vi "Lab2-InstructorHint-Calc-DisplayOnly.vi"() -> ()   [LabVIEW 2018]
panel:
  out "DegFlag":bool
  in  "Tab Control":enum32{"Calculator", "Settings", "Debug"}(tab)
  in  "Calc Pad Cluster":T1
  out "Calc Display":string
  out "Mode":string
  in  "ButtonPropertiesArray":T2(array[cluster])=[{"On/off"=FALSE, "Character"="C", "Op?"=FALSE}, {"On/off"=FALSE, "Character"="sin", "Op?"=FALSE}, {"On/off"=FALSE, "Character"="cos", "Op?"=FALSE}, {"On/off"=FALSE, "Character"="Del", "Op?"=FALSE}, {"On/off"=FALSE, "Character"="+", "Op?"=FALSE}, {"On/off"=FALSE, "Character"="7", "Op?"=FALSE}, {"On/off"=FALSE, "Character"="8", "Op?"=FALSE}, {"On/off"=FALSE, "Character"="9", "Op?"=FALSE}, {"On/off"=FALSE, "Character"="-", "Op?"=FALSE}, {"On/off"=FALSE, "Character"="4", "Op?"=FALSE}, {"On/off"=FALSE, "Character"="5", "Op?"=FALSE}, {"On/off"=FALSE, "Character"="6", "Op?"=FALSE}, {"On/off"=FALSE, "Character"="*", "Op?"=FALSE}, {"On/off"=FALSE, "Character"="1", "Op?"=FALSE}, {"On/off"=FALSE, "Character"="2", "Op?"=FALSE}, {"On/off"=FALSE, "Character"="3", "Op?"=FALSE}, {"On/off"=FALSE, "Character"="/", "Op?"=FALSE}, {"On/off"=FALSE, "Character"="(", "Op?"=FALSE}, {"On/off"=FALSE, "Character"=")", "Op?"=FALSE}, {"On/off"=FALSE, "Character"="=", "Op?"=FALSE}, {"On/off"=FALSE, "Character"=".", "Op?"=FALSE}, {"On/off"=FALSE, "Character"="Equation", "Op?"=FALSE}, {"On/off"=FALSE, "Character"="^", "Op?"=FALSE}, {"On/off"=FALSE, "Character"="0", "Op?"=FALSE}, {"On/off"=FALSE, "Character"="tan", "Op?"=FALSE}, {"On/off"=FALSE, "Character"="exit", "Op?"=FALSE}, {"On/off"=FALSE, "Character"="Rad", "Op?"=FALSE}]
  out "ButtonIndex":i32[](array[numeric])
  out "ButtonChars":string[](array[string])
  out "KeyPressedStatus":bool[](array[boolean])
  out "c":dbl
  out "b":dbl
  out "a":dbl
  out "EqState":dbl
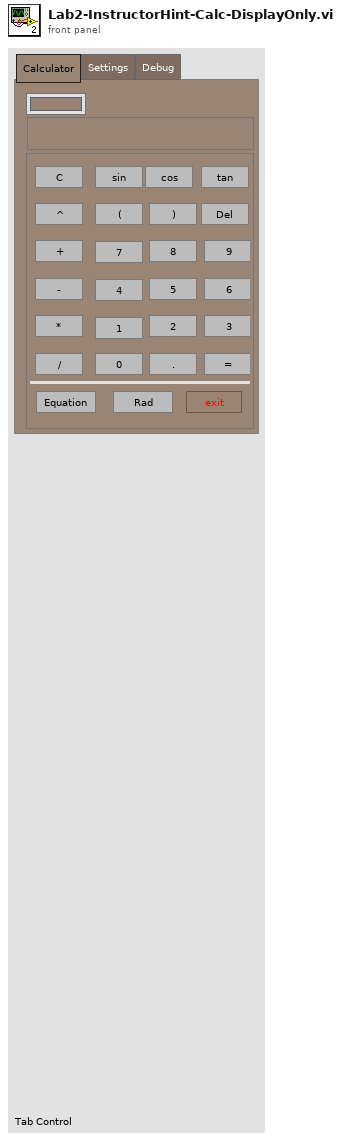
[diagram p1: front panel]
types:
  T1 = cluster{"B 0":bool, "B 1":bool, "B 2":bool, "B 3":bool, "B 4":bool, "B 5":bool, "B 6":bool, "B 7":bool, "B 8":bool, "B 9":bool, "B 10":bool, "B 11":bool, "B 12":bool, "B 13":bool, "B 14":bool, "B 15":bool, "B 16":bool, "B 17":bool, "B 18":bool, "B 19":bool, "B 20":bool, "B 21":bool, "B 22":bool, "B 23":bool, "B 24":bool, "Exit":bool, "B 25":bool}
  T2 = cluster{"On/off":bool, "Character":string, "Op?":bool}[]
  T3 = cluster{"On/off":bool, "Character":string, "Op?":bool}
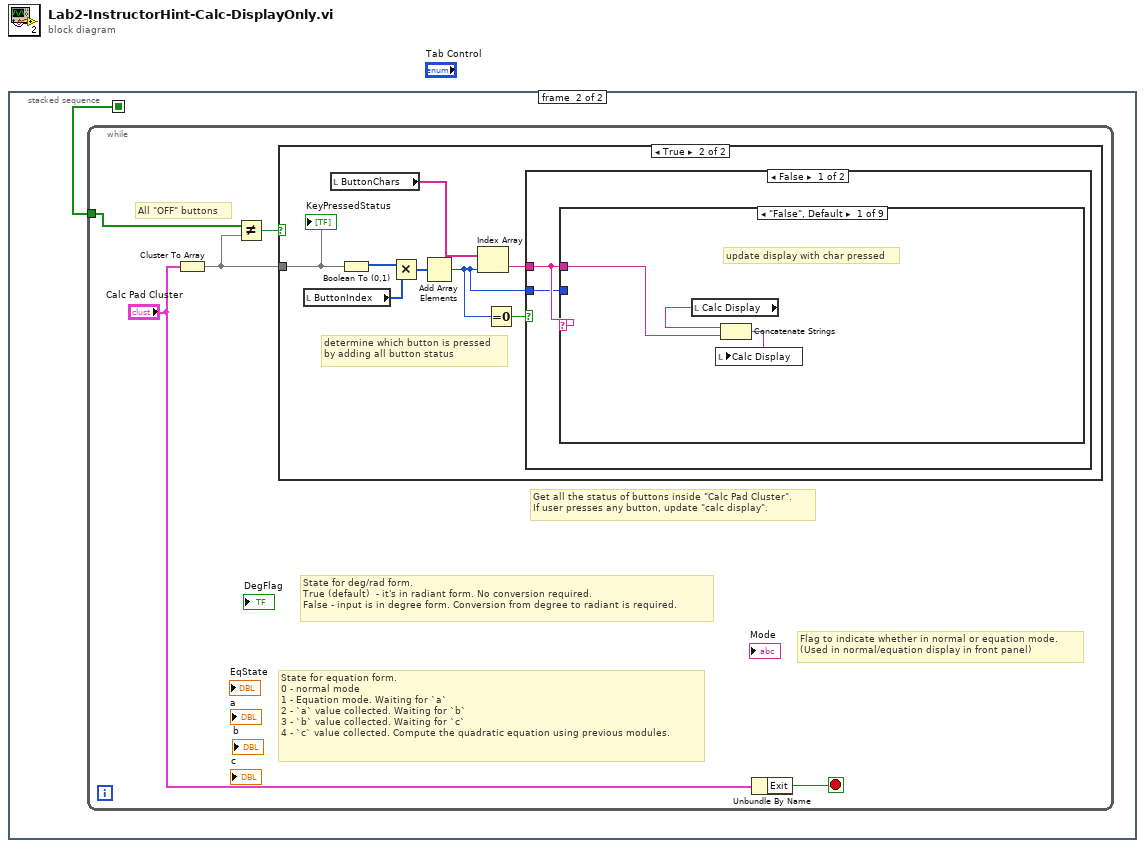
[diagram p0: block diagram]
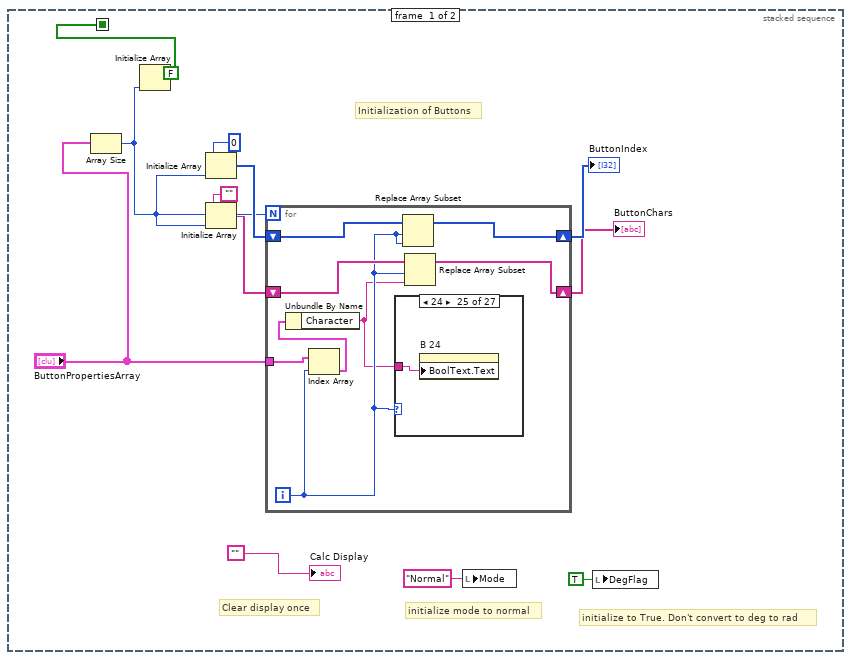
[diagram p2: hidden frame]
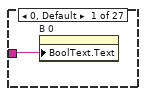
[diagram p3: hidden frame]
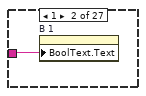
[diagram p4: hidden frame]
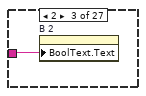
[diagram p5: hidden frame]
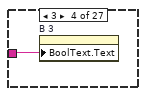
[diagram p6: hidden frame]
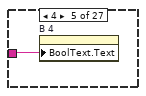
[diagram p7: hidden frame]
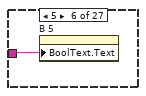
[diagram p8: hidden frame]
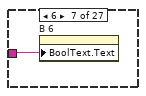
[diagram p9: hidden frame]
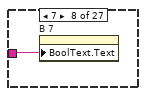
[diagram p10: hidden frame]
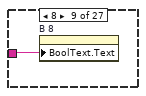
[diagram p11: hidden frame]
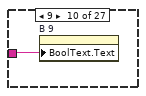
[diagram p12: hidden frame]
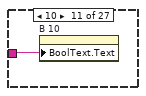
[diagram p13: hidden frame]
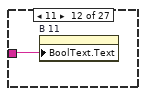
[diagram p14: hidden frame]
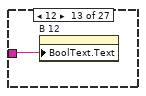
[diagram p15: hidden frame]
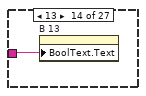
[diagram p16: hidden frame]
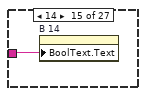
[diagram p17: hidden frame]
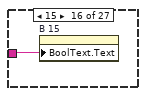
[diagram p18: hidden frame]
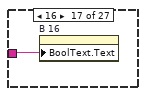
[diagram p19: hidden frame]
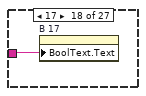
[diagram p20: hidden frame]
diagram:
  n1 = stacked-sequence {
    seq-local: [w12 _] -> [_ w49]
    frame #0 {
      # "initialize to True. Don't convert to deg to rad"
      # "initialize mode to normal"
      # "Clear display once"
      # "Initialization of Buttons"
      n2 = Array Size(array="ButtonPropertiesArray") -> (size(s)=w6:i32)
      n3 = Initialize Array(FALSE, w6) -> (w12:bool[])
      n4 = Initialize Array(0, w6) -> (w9:i32[])
      n5 = Initialize Array("", w6) -> (w5:string[])
      n6 = for {
        N: w6 -> [_]
        tunnel: "ButtonPropertiesArray" -> [w17]
        shift-right: [w20] -> w8
        shift-left: w9 -> [w21]
        shift-right: [w16] -> w4
        shift-left: w5 -> [w19]
        i -> [w15]
        n7 = Index Array(array=w17, index=w15) -> (element=w18:T3)
        n8 = Unbundle By Name(w18) -> ("Character"=w14:string)
        n9 = case shown="24" w15 {
          tunnel: w14 -> [w22 w23 w24 w25 w26 w27 w28 w29 w30 w31 w32 w33 w34 w35 w36 w37 w38 w39 w40 w41 w42 w43 w44 w45 w46 w47 w48]
          frame 0, Default {
            n10 = property on="B 0" class="Bool"("BoolText.Text"=w22) -> ()  [unwired: 2 in, 2 out]
          }
          frame 1 {
            n11 = property on="B 1" class="Bool"("BoolText.Text"=w23) -> ()  [unwired: 2 in, 2 out]
          }
          frame 2 {
            n12 = property on="B 2" class="Bool"("BoolText.Text"=w24) -> ()  [unwired: 2 in, 2 out]
          }
          frame 3 {
            n13 = property on="B 3" class="Bool"("BoolText.Text"=w25) -> ()  [unwired: 2 in, 2 out]
          }
          frame 4 {
            n14 = property on="B 4" class="Bool"("BoolText.Text"=w26) -> ()  [unwired: 2 in, 2 out]
          }
          frame 5 {
            n15 = property on="B 5" class="Bool"("BoolText.Text"=w27) -> ()  [unwired: 2 in, 2 out]
          }
          frame 6 {
            n16 = property on="B 6" class="Bool"("BoolText.Text"=w28) -> ()  [unwired: 2 in, 2 out]
          }
          frame 7 {
            n17 = property on="B 7" class="Bool"("BoolText.Text"=w29) -> ()  [unwired: 2 in, 2 out]
          }
          frame 8 {
            n18 = property on="B 8" class="Bool"("BoolText.Text"=w30) -> ()  [unwired: 2 in, 2 out]
          }
          frame 9 {
            n19 = property on="B 9" class="Bool"("BoolText.Text"=w31) -> ()  [unwired: 2 in, 2 out]
          }
          frame 10 {
            n20 = property on="B 10" class="Bool"("BoolText.Text"=w32) -> ()  [unwired: 2 in, 2 out]
          }
          frame 11 {
            n21 = property on="B 11" class="Bool"("BoolText.Text"=w33) -> ()  [unwired: 2 in, 2 out]
          }
          frame 12 {
            n22 = property on="B 12" class="Bool"("BoolText.Text"=w34) -> ()  [unwired: 2 in, 2 out]
          }
          frame 13 {
            n23 = property on="B 13" class="Bool"("BoolText.Text"=w35) -> ()  [unwired: 2 in, 2 out]
          }
          frame 14 {
            n24 = property on="B 14" class="Bool"("BoolText.Text"=w36) -> ()  [unwired: 2 in, 2 out]
          }
          frame 15 {
            n25 = property on="B 15" class="Bool"("BoolText.Text"=w37) -> ()  [unwired: 2 in, 2 out]
          }
          frame 16 {
            n26 = property on="B 16" class="Bool"("BoolText.Text"=w38) -> ()  [unwired: 2 in, 2 out]
          }
          frame 17 {
            n27 = property on="B 17" class="Bool"("BoolText.Text"=w39) -> ()  [unwired: 2 in, 2 out]
          }
          frame 18 {
            n28 = property on="B 18" class="Bool"("BoolText.Text"=w40) -> ()  [unwired: 2 in, 2 out]
          }
          frame 19 {
            n29 = property on="B 19" class="Bool"("BoolText.Text"=w41) -> ()  [unwired: 2 in, 2 out]
          }
          frame 20 {
            n30 = property on="B 20" class="Bool"("BoolText.Text"=w42) -> ()  [unwired: 2 in, 2 out]
          }
          frame 21 {
            n31 = property on="B 21" class="Bool"("BoolText.Text"=w43) -> ()  [unwired: 2 in, 2 out]
          }
          frame 22 {
            n32 = property on="B 22" class="Bool"("BoolText.Text"=w44) -> ()  [unwired: 2 in, 2 out]
          }
          frame 23 {
            n33 = property on="B 23" class="Bool"("BoolText.Text"=w45) -> ()  [unwired: 2 in, 2 out]
          }
          frame 24 {
            n34 = property on="B 24" class="Bool"("BoolText.Text"=w46) -> ()  [unwired: 2 in, 2 out]
          }
          frame 25 {
            n35 = property on="Exit" class="Bool"("BoolText.Text"=w47) -> ()  [unwired: 2 in, 2 out]
          }
          frame 26 {
            n36 = property on="B 25" class="Bool"("BoolText.Text"=w48) -> ()  [unwired: 2 in, 2 out]
          }
        }
        n37 = Replace Array Subset(array=w21, new element=w15, index=w15) -> (w20:i32[])
        n38 = Replace Array Subset(array=w19, new element=w14, index=w15) -> (w16:string[])
      }
      "ButtonIndex" <- w8
      "ButtonChars" <- w4
      n39 = local write "Mode"("Normal" ("Mode")) -> ()
      n40 = local write "DegFlag"(TRUE ("DegFlag")) -> ()
      "Calc Display" <- ""
    }
    frame #1 {
      n41 = while {
        tunnel: w49 -> [w52]
        stop <- w50 stop-if-true
        # "Flag to indicate whether in normal or equation mode.\n(Used in normal/equation display in front panel)"
        # "State for deg/rad form.\nTrue (default)  - it's in radiant form. No conversion required.\nFalse - input is in degree form. Conversion from degree to radiant is required."
        # "State for equation form. \n0 - normal mode\n1 - Equation mode. Waiting for `a`\n2 - `a` value collected. Waiting for `b`\n3 - `b` value collected. Waiting for `c`\n4 - `c` value collected. Compute the quadratic equation using previous modules."
        # "Get all the status of buttons inside \"Calc Pad Cluster\".\nIf user presses any button, update \"calc display\"."
        # "All \"OFF\" buttons"
        n42 = Cluster To Array(cluster="Calc Pad Cluster") -> (array=w53:bool[])
        n43 = Not Equal?(x=w52, y=w53) -> (x != y?=w54:bool)
        n44 = case shown="True" w54 {
          tunnel: w53 -> [_ w57]
          frame False {
            # "no button is pressed"
          }
          frame True {
            # "determine which button is pressed\nby adding all button status"
            n45 = local read "ButtonIndex"() -> (w61:i32[])
            n46 = local read "ButtonChars"() -> (w59:string[])
            n47 = Boolean To (0,1)(Boolean=w57) -> (0, 1=w62:i16[])
            n48 = Multiply(x=w62, y=w61) -> (x*y=w60:i32[])
            n49 = Add Array Elements(numeric array=w60) -> (sum=w55:i32)
            n50 = Index Array(array=w59, index=w55) -> (element=w58:string)
            n51 = Equal To 0?(x=w55) -> (x = 0?=w56:bool)
            n52 = case shown="False" w56 {
              tunnel: w58 -> [w64 _]
              tunnel: w55 -> [w63 _]
              frame False {
                n53 = case shown="\"False\", Default" w64 {
                  tunnel: w64 -> [w66 _ _ w101 w104 w108 _ _ _]
                  tunnel: w63 -> [_ _ _ _ _ _ _ w116 w122]
                  frame "False", Default {
                    # "update display with char pressed"
                    n54 = local read "Calc Display"() -> (w67:string)
                    n55 = Concatenate Strings(w67, w66) -> (w65:string)
                    n56 = local write "Calc Display"(w65) -> ()
                  }
                  frame "=" {
                    n57 = local read "EqState"() -> (w68:dbl)
                    n58 = case shown="3" w68 {
                      frame 0, Default {
                        # "DegFlag is used to indicate whether \ncurrent string is in degree or radiant\nform"
                        n59 = local read "DegFlag"() -> (w70:bool)
                        n60 = local read "Calc Display"() -> (w71:string)
                        n61 = call "CalculateInputString_v2.vi"("Rad"=w70, "InputString"=w71) -> ("result"=w69:dbl)
                        n62 = Number To Fractional String(number=w69) -> (F-format string=w72:string)  [unwired: 3 in]
                        n63 = local write "Calc Display"(w72) -> ()
                      }
                      frame 1 {
                        n64 = flat-sequence {
                          frame #0 {
                            n65 = local read "Calc Display"() -> (w75:string)
                            n66 = Fract/Exp String To Number(string=w75) -> (number=w74:dbl)  [unwired: 3 in, 1 out]
                            n67 = local write "a"(w74) -> ()
                            n68 = local write "EqState"(2.0 ("EqFlag")) -> ()
                          }
                          frame #1 {
                            n69 = local write "Calc Display"("" ("Calc Display")) -> ()
                          }
                        }
                      }
                      frame 2 {
                        n70 = flat-sequence {
                          frame #0 {
                            n71 = local read "Calc Display"() -> (w79:string)
                            n72 = Fract/Exp String To Number(string=w79) -> (number=w78:dbl)  [unwired: 3 in, 1 out]
                            n73 = local write "b"(w78) -> ()
                            n74 = local write "EqState"(3.0 ("EqFlag")) -> ()
                          }
                          frame #1 {
                            n75 = local write "Calc Display"("" ("Calc Display")) -> ()
                          }
                        }
                      }
                      frame 3 {
                        # "change mode back\nto normal"
                        n76 = local write "Mode"("normal" ("Mode")) -> ()
                        n77 = local read "Calc Display"() -> (w94:string)
                        n78 = Fract/Exp String To Number(string=w94) -> (number=w93:dbl)  [unwired: 3 in, 1 out]
                        n79 = local write "c"(w93) -> ()
                        n80 = local read "c"() -> (w84:dbl)
                        n81 = local read "b"() -> (w85:dbl)
                        n82 = local read "a"() -> (w86:dbl)
                        n83 = local write "EqState"(0.0 ("EqFlag")) -> ()
                        n84 = call "quadratic_eq_solve.vi"("C"=w84, "B"=w85, "A"=w86) -> ("x2"=w82:dbl, "x1"=w83:dbl)
                        n85 = Number To Fractional String(number=w83) -> (F-format string=w90:string)  [unwired: 3 in]
                        n86 = Number To Fractional String(number=w82) -> (F-format string=w89:string)  [unwired: 3 in]
                        n87 = Concatenate Strings("x1=" ("string"), w90, "x2=" ("string"), w89) -> (w87:string)
                        n88 = local write "Calc Display"(w87) -> ()
                      }
                    }
                  }
                  frame "Del" {
                    n89 = local read "Calc Display"() -> (w98:string)
                    n90 = String Length(string=w98) -> (length=w97:i32)
                    n91 = Decrement(x=w97) -> (x-1=w96:i32)
                    n92 = Replace Substring(2:w96, 5:w98) -> (0:w95:string)  [unwired: 2 in, 1 out]
                    n93 = local write "Calc Display"(w95) -> ()
                  }
                  frame "sin" {
                    n94 = local read "Calc Display"() -> (w102:string)
                    n95 = Concatenate Strings(w102, w101, "(" ("string")) -> (w99:string)
                    n96 = local write "Calc Display"(w99) -> ()
                  }
                  frame "cos" {
                    n97 = local read "Calc Display"() -> (w105:string)
                    n98 = Concatenate Strings(w105, w104, "(" ("string")) -> (w103:string)
                    n99 = local write "Calc Display"(w103) -> ()
                  }
                  frame "tan" {
                    n100 = local read "Calc Display"() -> (w109:string)
                    n101 = Concatenate Strings(w109, w108, "(" ("string")) -> (w107:string)
                    n102 = local write "Calc Display"(w107) -> ()
                  }
                  frame "Equation" {
                    n103 = local write "Calc Display"("" ("Calc Display")) -> ()
                    n104 = local write "EqState"(1.0 ("EqFlag")) -> ()
                    n105 = local write "Mode"("Equation" ("Mode")) -> ()
                  }
                  frame "Rad" {
                    w115 = "Deg" ("Boolean Text.Text")
                    # "Rad button is clicked. Change to Deg"
                    n106 = local write "DegFlag"(FALSE ("DegFlag")) -> ()
                    n107 = property on="B 25" class="Bool"("BoolText.Text"=w115) -> ()  [unwired: 2 in, 2 out]
                    n108 = local read "ButtonChars"() -> (w117:string[])
                    n109 = Replace Array Subset(array=w117, new element=w115, index=w116) -> (w114:string[])
                    n110 = local write "ButtonChars"(w114) -> ()
                  }
                  frame "Deg" {
                    w121 = "Rad" ("Boolean Text.Text")
                    # "Deg button is clicked. Change to Rad"
                    n111 = local write "DegFlag"(TRUE ("DegFlag")) -> ()
                    n112 = property on="B 25" class="Bool"("BoolText.Text"=w121) -> ()  [unwired: 2 in, 2 out]
                    n113 = local read "ButtonChars"() -> (w120:string[])
                    n114 = Replace Array Subset(array=w120, new element=w121, index=w122) -> (w119:string[])
                    n115 = local write "ButtonChars"(w119) -> ()
                  }
                }
              }
              frame True {
                # "When 'C' is pressed"
                n116 = local write "Calc Display"("" ("Calc Display")) -> ()
                n117 = local write "Mode"("Normal" ("Mode")) -> ()
                n118 = local write "EqState"(0.0 ("EqState")) -> ()
              }
            }
            "KeyPressedStatus" <- w57
          }
        }
        n119 = Unbundle By Name("Calc Pad Cluster") -> ("Exit"=w50:bool)
      }
    }
  }
